vi "CRYPlot Octave Graph.vi"(6 "sOption":string, 7 "pGraph VI In":refnum<vi>, 9 "Flattened Property":string, 10 "Flattened Scale Property":string, 11 "Selected Rows In":i32[](array[numeric])) -> (0 "Color Info":u32[](array[numeric]), 1 "Curve Name":string[](array[string]), 2 "All Rows Out":i32[](array[numeric]), 3 "ItemSyms":i32[](array[numeric]))   [LabVIEW 2013]
uses:
  CRYWindow/DataView/Control/CRYGraph Scale.ctl
panel:
  in  "Graph Scale Property":T1={"X Scale.Maximum"=0.0, "X Scale.Minimum"=0.0, "Y0 Scale.Maximum"=0.0, "Y0 Scale.Minimum"=0.0, "Y1 Scale.Maximum"=0.0, "Y1 Scale.Minimum"=0.0, "X Scale.MapMode"=2, "Y1 Scale.MapMode"=2, "Y0 Scale.MapMode"=2, "ScaleFitX"=FALSE, "ScaleFitY"=FALSE, "ScaleFitY 2"=FALSE}
  in  "Plot Settings":T2(array[cluster])
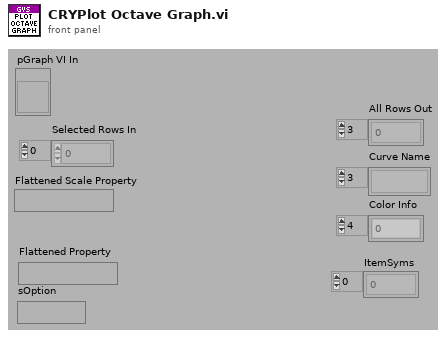
[diagram p1: front panel]
types:
  T1 = typedef "CRYGraph Scale.ctl" = cluster{"X Scale.Maximum":dbl, "X Scale.Minimum":dbl, "Y0 Scale.Maximum":dbl, "Y0 Scale.Minimum":dbl, "Y1 Scale.Maximum":dbl, "Y1 Scale.Minimum":dbl, "X Scale.MapMode":u8, "Y1 Scale.MapMode":u8, "Y0 Scale.MapMode":u8, "ScaleFitX":bool, "ScaleFitY":bool, "ScaleFitY 2":bool}
  T2 = cluster{"Color":u32, "Interpolation":u8, "Point Style":u8, "Line Style":u8, "Point Color":u32, "Line Width":u8, "Bar Plot Style":u8, "Fill To":i16}[]
  T3 = typedef "CRYData Cluster.ctl" = cluster{"Name":string, "Curve":cluster{"x":dbl, "y":dbl, "z":dbl}[], "X data":u16, "Y data":u16, "Z data":u16, "X axis":u16, "Y axis":u16, "Z axis":u16, "X unit":string, "Y unit":string, "Z unit":string, "X dB ref":dbl, "Y dB ref":dbl, "Z dB ref":dbl, "single val":bool, "protected":bool, "display X":bool, "display Y":bool, "display Z":bool, "Test Info":string, "Step No.":i32, "Plot Settings":cluster{"Color":u32, "Interpolation":u8, "Point Style":u8, "Line Style":u8, "Point Color":u32, "Line Width":u8, "Bar Plot Style":u8, "Fill To":i16}, "AutoProtect":bool}
  T4 = cluster{"Color":u32, "Interpolation":u8, "Point Style":u8, "Line Style":u8, "Point Color":u32, "Line Width":u8, "Bar Plot Style":u8, "Fill To":i16}
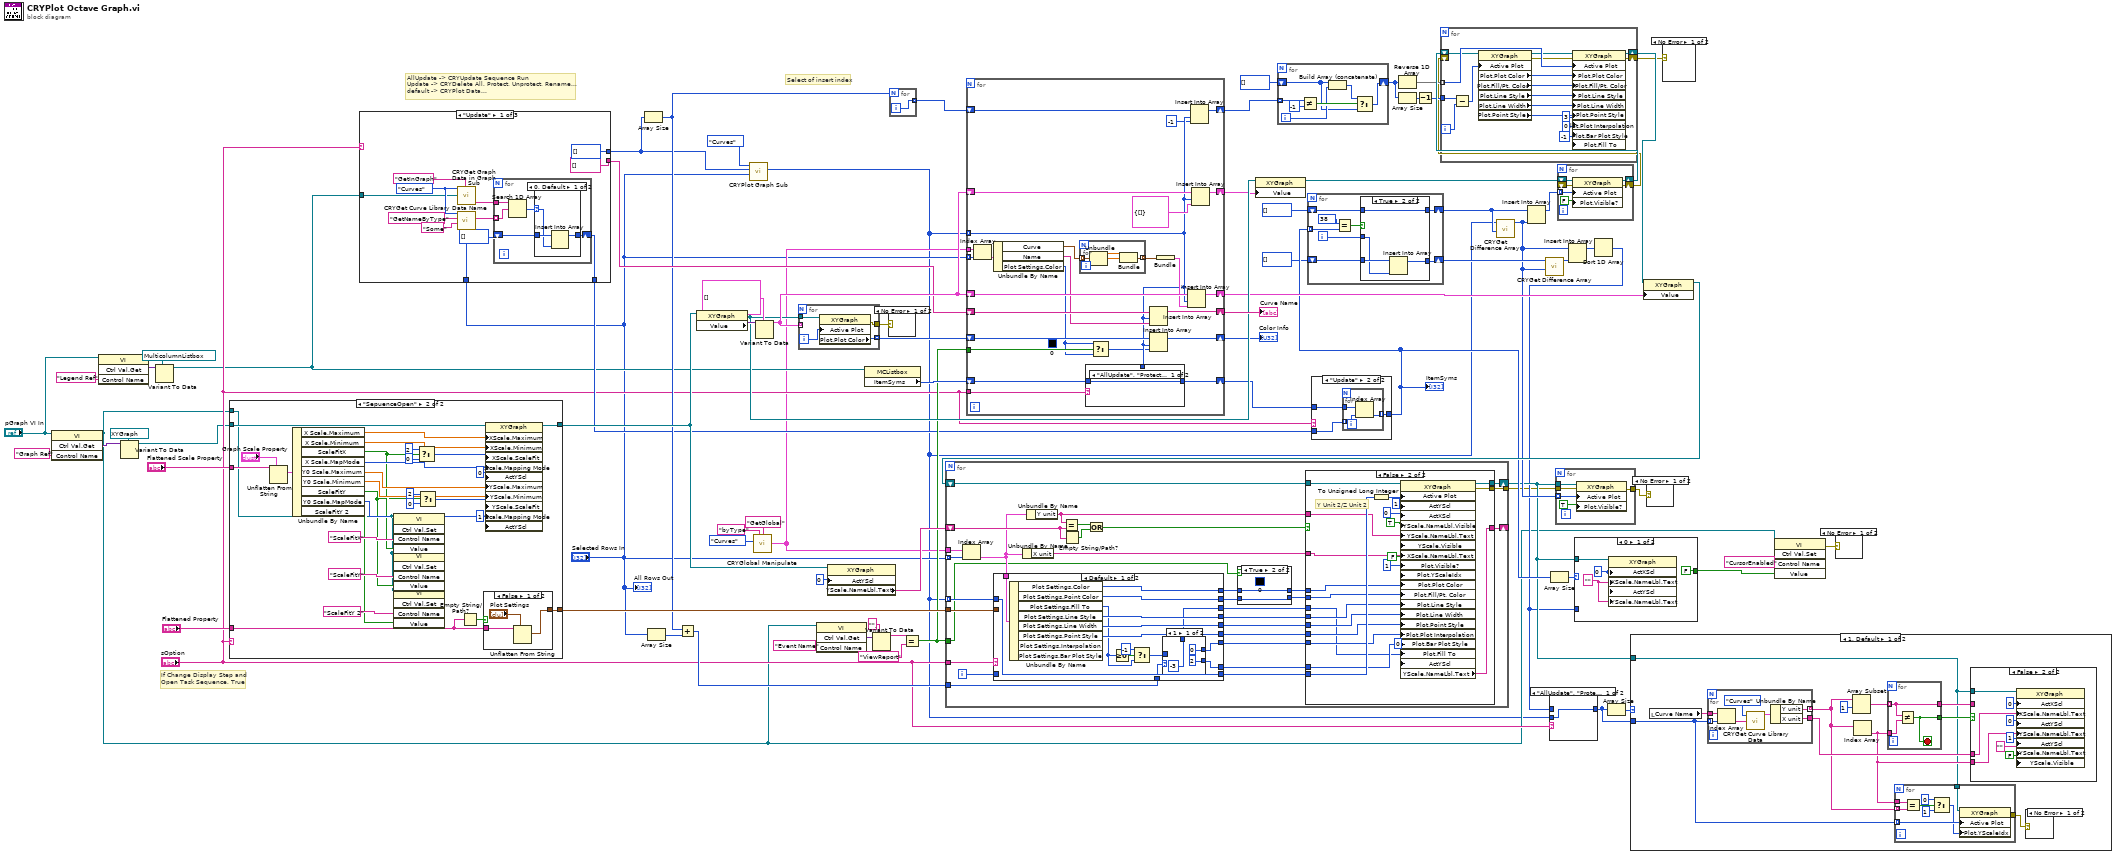
[diagram p0: block diagram]
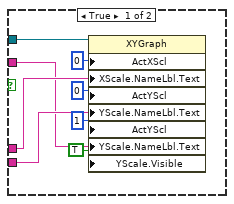
[diagram p7: hidden frame]
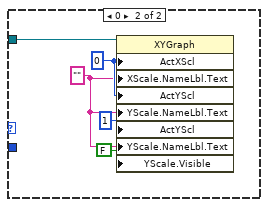
[diagram p8: hidden frame]
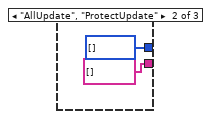
[diagram p11: hidden frame]
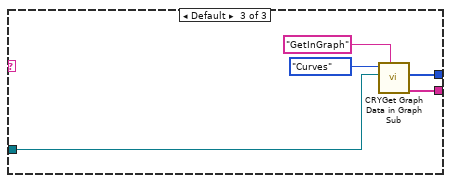
[diagram p12: hidden frame]
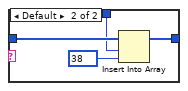
[diagram p13: hidden frame]
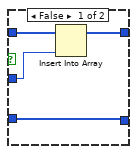
[diagram p15: hidden frame]
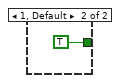
[diagram p16: hidden frame]
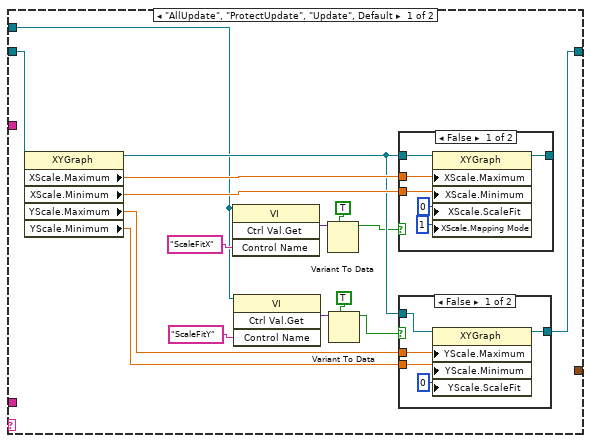
[diagram p17: hidden frame]
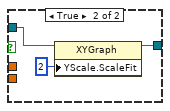
[diagram p18: hidden frame]
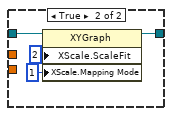
[diagram p19: hidden frame]
diagram:
  # "AllUpdate -> CRYUpdate Sequence Run\nUpdate -> CRYDelete All, Protect, Unprotect, Rename...\ndefault -> CRYPlot Data..."
  # "Select of insert index"
  # "If Change Display Step and \nOpen Task Sequence, True"
  n1 = invoke class="VI" method="Ctrl Val.Get"(reference="pGraph VI In", "Control Name"="Graph Ref") -> (reference out=w9:refnum<vi>, "Get Control Value Variant"=w13:variant)  [unwired: 2 in, 2 out]
  n2 = invoke class="VI" method="Ctrl Val.Get"(reference="pGraph VI In", "Control Name"="Legend Ref") -> ("Get Control Value Variant"=w17:variant)  [unwired: 2 in, 3 out]
  n3 = Variant To Data(type=refnum<vi> refnum ("XY Graph"), Variant=w13) -> (data=w12:refnum<vi>)  [unwired: 1 in, 1 out]
  n4 = Variant To Data(type=refnum<vi> refnum ("GMListbox"), Variant=w17) -> (data=w10:refnum<vi>)  [unwired: 1 in, 1 out]
  n5 = case shown="\"SepuenceOpen\"" "sOption" {
    tunnel: w12 -> [w96 w143]
    tunnel: [w91 w142] -> w59
    tunnel: "Flattened Scale Property" -> [_ w133]
    tunnel: [_ w129] -> w71
    tunnel: "Flattened Property" -> [_ w128]
    tunnel: w9 -> [w81 w115]
    frame "AllUpdate", "ProtectUpdate", "Update", Default {
      n6 = property class="XYGraph"(reference=w96) -> (reference out=w90:refnum<vi>, "XScale.Maximum"=w95:dbl, "XScale.Minimum"=w94:dbl, "YScale.Maximum"=w93:dbl, "YScale.Minimum"=w92:dbl)  [unwired: 1 in, 1 out]
      n7 = invoke class="VI" method="Ctrl Val.Get"(reference=w81, "Control Name"="ScaleFitX") -> ("Get Control Value Variant"=w85:variant)  [unwired: 2 in, 3 out]
      n8 = invoke class="VI" method="Ctrl Val.Get"(reference=w81, "Control Name"="ScaleFitY") -> ("Get Control Value Variant"=w88:variant)  [unwired: 2 in, 3 out]
      n9 = Variant To Data(type=TRUE, Variant=w85) -> (data=w83:bool)  [unwired: 1 in, 1 out]
      n10 = Variant To Data(type=TRUE, Variant=w88) -> (data=w82:bool)  [unwired: 1 in, 1 out]
      n11 = case shown="False" w83 {
        tunnel: w95 -> [w110 _]
        tunnel: w94 -> [w109 _]
        tunnel: w90 -> [w108 w114]
        tunnel: [w107 w113] -> _
        frame False {
          n12 = property class="XYGraph"(reference=w108, "XScale.Maximum"=w110, "XScale.Minimum"=w109, "XScale.ScaleFit"=u8 0 ("X Scale.Scale Fit"), "XScale.Mapping Mode"=u8 1 ("X Scale.Mapping Mode")) -> (reference out=w107:refnum<vi>)  [unwired: 1 in, 1 out]
        }
        frame True {
          n13 = property class="XYGraph"(reference=w114, "XScale.ScaleFit"=u8 2 ("X Scale.Scale Fit"), "XScale.Mapping Mode"=u8 1 ("X Scale.Mapping Mode")) -> (reference out=w113:refnum<vi>)  [unwired: 1 in, 1 out]
        }
      }
      n14 = case shown="False" w82 {
        tunnel: w90 -> [w101 w104]
        tunnel: [w100 w103] -> w91
        tunnel: w93 -> [w99 _]
        tunnel: w92 -> [w98 _]
        frame False {
          n15 = property class="XYGraph"(reference=w101, "YScale.Maximum"=w99, "YScale.Minimum"=w98, "YScale.ScaleFit"=u8 0 ("Y Scale.Scale Fit")) -> (reference out=w100:refnum<vi>)  [unwired: 1 in, 1 out]
        }
        frame True {
          n16 = property class="XYGraph"(reference=w104, "YScale.ScaleFit"=u8 2 ("Y Scale.Scale Fit")) -> (reference out=w103:refnum<vi>)  [unwired: 1 in, 1 out]
        }
      }
    }
    frame "SepuenceOpen" {
      n17 = Unflatten From String(type="Graph Scale Property", binary string=w133) -> (value=w132:T1)  [unwired: 3 in, 2 out]
      n18 = Unbundle By Name(w132) -> ("X Scale.Maximum"=w139:dbl, "X Scale.Minimum"=w138:dbl, "ScaleFitX"=w118:bool, "X Scale.MapMode"=w135:u8, "Y0 Scale.Maximum"=w137:dbl, "Y0 Scale.Minimum"=w136:dbl, "ScaleFitY"=w117:bool, "Y0 Scale.MapMode"=w134:u8, "ScaleFitY 2"=w116:bool)
      n19 = invoke class="VI" method="Ctrl Val.Set"(reference=w115, "Control Name"="ScaleFitX", "Value"=w118) -> ()  [unwired: 2 in, 5 out]
      n20 = invoke class="VI" method="Ctrl Val.Set"(reference=w115, "Control Name"="ScaleFitY", "Value"=w117) -> ()  [unwired: 2 in, 5 out]
      n21 = invoke class="VI" method="Ctrl Val.Set"(reference=w115, "Control Name"="ScaleFitY 2", "Value"=w116) -> ()  [unwired: 2 in, 5 out]
      n22 = Select(t=u8 2, s=w118, f=u8 0 ("X Scale.Scale Fit")) -> (s? t:f=w123:u8)
      n23 = Select(t=u8 2, s=w117, f=u8 0 ("X Scale.Scale Fit")) -> (s? t:f=w122:u8)
      n24 = Empty String/Path?(string/path=w128) -> (empty?=w130:bool)
      n25 = case shown="False" w130 {
        tunnel: w128 -> [w146 _]
        tunnel: [w144 _] -> w129
        frame False {
          n26 = Unflatten From String(type="Plot Settings", binary string=w146) -> (value=w144:T2)  [unwired: 3 in, 2 out]
        }
        frame True {
        }
      }
      n27 = property class="XYGraph"(reference=w143, "XScale.Maximum"=w139, "XScale.Minimum"=w138, "XScale.ScaleFit"=w123, "XScale.Mapping Mode"=w135, "ActYScl"=0 ("Active Y Scale"), "YScale.Maximum"=w137, "YScale.Minimum"=w136, "YScale.ScaleFit"=w122, "YScale.Mapping Mode"=w134, "ActYScl"=1 ("Active Y Scale")) -> (reference out=w142:refnum<vi>)  [unwired: 1 in, 1 out]
    }
  }
  n28 = case shown="\"Update\"" "sOption" {
    tunnel: [string[] [] ("Names Out") string[] [] ("Names Out") w174] -> w69
    tunnel: [i32[] [] ("Rows") i32[] [] ("Rows") w171] -> w3
    tunnel: "Selected Rows In" -> [w149 _ _]
    tunnel: [w148 _ _] -> w34
    tunnel: w10 -> [w147 _ w170]
    frame "Update" {
      w151 = enum16{"Curves", "Values", "Results", "WFM"}."Curves" ("Type")
      n29 = call "CRYGet Curve Library Data Name.vi"("nData"=w149, "sOption"="Some", "sAction"="GetNameByType", "Type"=w151) -> ("sNames"=w155:string[])  [unwired: 4 in, 3 out]
      n30 = call "CRYGet Graph Data in Graph Sub.vi"("sOption"="GetInGraph", "Legend Refnum"=w147, "Type In"=w151) -> ("Names Out"=w154:string[])  [unwired: 4 in, 4 out]
      n31 = for {
        tunnel: w154 -> [w160]
        tunnel: w155 -> [w159] mode=indexing
        shift-right: [w161] -> w148
        shift-left: i32[] [] -> [w162]
        n32 = Search 1D Array(1D array=w160, element=w159) -> (index of element=w163:i32)  [unwired: 1 in]
        n33 = case shown="0, Default" w163 {
          selector: w163 -> [w164 _]
          tunnel: w162 -> [w166 w167]
          tunnel: [w165 w167] -> w161
          frame 0, Default {
            n34 = Insert Into Array(array=w166, new element=w164) -> (w165:i32[])  [unwired: 1 in]
          }
          frame -1 {
          }
        }
      }
    }
    frame "AllUpdate", "ProtectUpdate" {
    }
    frame Default {
      n35 = call "CRYGet Graph Data in Graph Sub.vi"("sOption"="GetInGraph", "Legend Refnum"=w170, "Type In"=enum16{"Curves", "Values", "Results", "WFM"}."Curves" ("Type")) -> ("Names Out"=w174:string[], "Rows"=w171:i32[])  [unwired: 4 in, 3 out]
    }
  }
  n36 = Array Size(array=w3) -> (size(s)=w39:i32)
  n37 = Array Size(array="Selected Rows In") -> (size(s)=w40:i32)
  n38 = Add(x=w39, y=w40) -> (x+y=w38:i32)
  n39 = property class="XYGraph"(reference=w59) -> (reference out=w67:refnum<vi>, "Value"=w77:variant)  [unwired: 1 in, 1 out]
  n40 = call "CRYPlot Graph Sub.vi"("nData2 In"="Selected Rows In", "nData1 In"=w3, "Type"=enum16{"Curves", "Values", "Results", "WFM"}."Curves") -> ("nData Out"=w1:i32[])  [unwired: 8 in]
  n41 = call "CRYGlobal Manipulate.vi"("Type"=enum16{"Curves", "Values", "Results", "WFM"}."Curves", "sOption"="byType", "sAction"="GetGlobal") -> ("Curves Out"=w5:T3[])  [unwired: 6 in, 6 out]
  n42 = Variant To Data(type=cluster{cluster{"x":dbl, "z":dbl}[]}[] [], Variant=w77) -> (data=w76:cluster{cluster{"x":dbl, "z":dbl}[]}[])  [unwired: 1 in, 1 out]
  n43 = for {
    tunnel: w76 -> [_] mode=indexing
    tunnel: w67 -> [w178]
    tunnel: [w177] -> w75 mode=indexing
    tunnel: [w175] -> w20
    i -> [w176]
    n44 = property class="XYGraph"(reference=w178, "Active Plot"=w176) -> (error out=w175:errorcluster, "Plot.Plot Color"=w177:u32)  [unwired: 1 in, 1 out]
  }
  n45 = invoke class="VI" method="Ctrl Val.Get"(reference=w9, "Control Name"="Event Name") -> ("Get Control Value Variant"=w46:variant)  [unwired: 2 in, 3 out]
  n46 = property class="XYGraph"(reference=w59, "ActYScl"=0 ("Active Y Scale")) -> ("YScale.NameLbl.Text"=w60:string)  [unwired: 1 in, 2 out]
  n47 = property class="MCListbox"(reference=w10) -> ("ItemSyms"=w63:i32[])  [unwired: 1 in, 2 out]
  n48 = Variant To Data(type="" ("Control Name"), Variant=w46) -> (data=w44:string)  [unwired: 1 in, 1 out]
  n49 = case shown="No Error" w20 {
    frame No Error {
    }
    frame Error {
    }
  }
  n50 = for {
    N: w39 -> [_]
    tunnel: [w179] -> w57 mode=indexing
    i -> [w179]
  }
  n51 = Equal?(x=w44, y="ViewReport" ("regular expression")) -> (x = y?=w42:bool)
  n52 = for {
    tunnel: w5 -> [w205]
    tunnel: "Selected Rows In" -> [w202] mode=indexing
    shift-right: [w203] -> w65
    shift-left: w76 -> [w204]
    tunnel: w1 -> [w185] mode=indexing
    shift-right: [w193] -> w74
    shift-left: w69 -> [w197]
    shift-right: [w194] -> w41
    shift-left: w75 -> [w195]
    shift-right: [w191] -> w64
    shift-left: w76 -> [w190]
    shift-right: [w188] -> w35
    shift-left: w63 -> [w189]
    shift-right: [w186] -> w56
    shift-left: w57 -> [w187]
    tunnel: w42 -> [w183]
    tunnel: "sOption" -> [w181]
    (unwired) u32 0
    n53 = Index Array(array=w205, index=w202) -> (element=w199:T3)
    n54 = Unbundle By Name(w199) -> ("Curve"=w200:cluster{"x":dbl, "y":dbl, "z":dbl}[], "Name"=w196:string, "Plot Settings.Color"=w180:u32)
    n55 = for {
      tunnel: w200 -> [w213] mode=indexing
      tunnel: [w212] -> w201 mode=indexing
      n56 = Unbundle(w213) -> ("x"=w211:dbl, "y"=w214:dbl)  [unwired: 1 out]
      n57 = Bundle("x"=w211, "y"=w214) -> (w212:cluster{"x":dbl, "y":dbl})  [unwired: 1 out]
    }
    n58 = case shown="\"AllUpdate\", \"ProtectUpdate\", \"Update\"" w181 {
      tunnel: w189 -> [w206 w210]
      tunnel: [w206 w209] -> w188
      tunnel: w185 -> [_ w207]
      frame "AllUpdate", "ProtectUpdate", "Update" {
      }
      frame Default {
        n59 = Insert Into Array(array=w210, index=w207, new element=38) -> (w209:i32[])
      }
    }
    n60 = Select(t=w180, s=w183, f=w180) -> (s? t:f=w182:u32)
    n61 = Insert Into Array(array=w197, index=w185, new element=w196) -> (w193:string[])
    n62 = Insert Into Array(array=w195, index=w185, new element=w182) -> (w194:u32[])
    n63 = Bundle(w201) -> (w198:cluster{cluster{"x":dbl, "y":dbl}[]})  [unwired: 1 in]
    n64 = Insert Into Array(array=w204, index=w185, new element=w198) -> (w203:cluster{cluster{"x":dbl, "z":dbl}[]}[])
    n65 = Insert Into Array(array=w187, index=w185, new element=-1 ("new element/subarray")) -> (w186:i32[])
    n66 = Insert Into Array(array=w190, index=w185, new element=cluster{cluster{"x":dbl, "y":dbl}[]} {[]} ("output cluster")) -> (w191:cluster{cluster{"x":dbl, "z":dbl}[]}[])
  }
  "Curve Name" <- w74
  "Color Info" <- w41
  n67 = property class="XYGraph"(reference=w67, "Value"=w64) -> (reference out=w66:refnum<vi>)  [unwired: 1 in, 1 out]
  n68 = for {
    tunnel: w56 -> [w221] mode=indexing
    shift-right: [w217] -> w51
    shift-left: i32[] [] ("Selected Rows In") -> [w215]
    i -> [w216]
    n69 = Not Equal?(x=w221, y=-1) -> (x != y?=w219:bool)
    n70 = Build Array (concatenate)(w215, w216) -> (w218:i32[])
    n71 = Select(t=w218, s=w219, f=w215) -> (s? t:f=w217:i32[])
  }
  n72 = case shown="\"Update\"" "sOption" {
    tunnel: w34 -> [_ w224]
    tunnel: w35 -> [w222 w225]
    tunnel: [w222 w223] -> w33
    frame Default {
    }
    frame "Update" {
      n73 = for {
        tunnel: w225 -> [w228]
        tunnel: w224 -> [w227] mode=indexing
        tunnel: [w226] -> w223 mode=indexing
        n74 = Index Array(array=w228, index=w227) -> (element=w226:i32)
      }
    }
  }
  "ItemSyms" <- w33
  n75 = for {
    tunnel: w33 -> [w235] mode=indexing
    shift-right: [w234] -> w37
    shift-left: i32[] [] ("Selected Rows In") -> [w233]
    shift-right: [w229] -> w29
    shift-left: i32[] [] ("Selected Rows In") -> [w230]
    i -> [w232]
    n76 = Equal?(x=38, y=w235) -> (x = y?=w231:bool)
    n77 = case shown="True" w231 {
      tunnel: [w239 w241] -> w234
      tunnel: w233 -> [w240 w241]
      tunnel: w232 -> [w238 w242]
      tunnel: w230 -> [w237 w244]
      tunnel: [w237 w243] -> w229
      frame False {
        n78 = Insert Into Array(array=w240, new element=w238) -> (w239:i32[])  [unwired: 1 in]
      }
      frame True {
        n79 = Insert Into Array(array=w244, new element=w242) -> (w243:i32[])  [unwired: 1 in]
      }
    }
  }
  n80 = Reverse 1D Array(array=w51) -> (reversed array=w52:i32[])
  n81 = Array Size(array=w51) -> (size(s)=w50:i32)
  n82 = Decrement(x=w50) -> (x-1=w49:i32)
  n83 = call "CRYGet Difference Array.vi"("Array 2"=w37, "Array 1"=w1) -> ("Diff Out"=w28:i32[])  [unwired: 8 in, 1 out]
  n84 = Insert Into Array(array=w37, new element=w28) -> (w58:i32[])  [unwired: 1 in]
  n85 = call "CRYGet Difference Array.vi"("Array 2"=w28, "Array 1"=w29) -> ("Diff Out"=w31:i32[])  [unwired: 8 in, 1 out]
  n86 = Array Size(array=w33) -> (size(s)=w80:i32)
  n87 = for {
    shift-right: [w248] -> w54
    shift-left: w66 -> [w250]
    tunnel: w58 -> [w247] mode=indexing
    shift-right: [w246] -> w36
    shift-left: _ -> [w245]
    n88 = property class="XYGraph"(reference=w250, error in=w245, "Active Plot"=w247, "Plot.Visible?"=FALSE ("Plot.Visible")) -> (reference out=w248:refnum<vi>, error out=w246:errorcluster)
  }
  n89 = for {
    tunnel: w52 -> [w262] mode=indexing
    shift-right: [w260] -> w53
    shift-left: w54 -> [w261]
    tunnel: w49 -> [w258]
    shift-right: [w254] -> w48
    shift-left: w36 -> [_]
    i -> [w257]
    n90 = Subtract(x=w258, y=w257) -> (x-y=w256:i32)
    n91 = property class="XYGraph"(reference=w261, "Active Plot"=w256) -> (reference out=w259:refnum<vi>, error out=w255:errorcluster, "Plot.Plot Color"=w267:u32, "Plot.Fill/Pt. Color"=w266:u32, "Plot.Line Style"=w265:u8, "Plot.Line Width"=w264:u8, "Plot.Point Style"=w263:u8)  [unwired: 1 in]
    n92 = property class="XYGraph"(reference=w259, error in=w255, "Active Plot"=w262, "Plot.Plot Color"=w267, "Plot.Fill/Pt. Color"=w266, "Plot.Line Style"=w265, "Plot.Line Width"=w264, "Plot.Point Style"=w263, "Plot.Plot Interpolation"=u8 3, "Plot.Bar Plot Style"=u8 0, "Plot.Fill To"=i16 -1) -> (reference out=w260:refnum<vi>, error out=w254:errorcluster)
  }
  n93 = Insert Into Array(array=w28, new element=w31) -> (w30:i32[])  [unwired: 1 in]
  n94 = Sort 1D Array(array=w30) -> (sorted array=w24:i32[])
  n95 = case shown="\"AllUpdate\", \"ProtectUpdate\", \"SepuenceOpen\"" "sOption" {
    tunnel: [w268 w269] -> w23
    tunnel: w1 -> [w268 _]
    tunnel: w24 -> [_ w269]
    frame "AllUpdate", "ProtectUpdate", "SepuenceOpen" {
    }
    frame Default {
    }
  }
  n96 = Array Size(array=w23) -> (size(s)=w27:i32)
  n97 = property class="XYGraph"(reference=w53, "Value"=w65) -> (reference out=w73:refnum<vi>)  [unwired: 1 in, 1 out]
  n98 = for {
    tunnel: "Selected Rows In" -> [w299] mode=indexing
    tunnel: w5 -> [w298]
    tunnel: w71 -> [w293]
    tunnel: "sOption" -> [w294]
    shift-right: [w295] -> w26
    shift-left: w73 -> [w283]
    tunnel: w1 -> [w282] mode=indexing
    shift-right: [w280] -> _
    shift-left: w60 -> [w286]
    tunnel: w42 -> [w278]
    tunnel: w38 -> [w271]
    tunnel: [w270] -> w19
    i -> [w287]
    n99 = Index Array(array=w298, index=w299) -> (element=w285:T3)
    n100 = case shown="Default" w294 {
      tunnel: w293 -> [_ w330]
      tunnel: [w318 w339] -> w277
      tunnel: [w317 w338] -> w275
      tunnel: [w305 w327] -> w292
      tunnel: [w316 w337] -> w291
      tunnel: [w315 w336] -> w290
      tunnel: [w314 w335] -> w289
      tunnel: [w307 w326] -> w288
      tunnel: w285 -> [w313 _]
      tunnel: w287 -> [_ w329]
      tunnel: [w309 w331] -> w281
      tunnel: w282 -> [w309 w331]
      tunnel: [w306 w325] -> w279
      tunnel: w271 -> [w308 _]
      frame Default {
        n101 = Unbundle By Name(w313) -> ("Plot Settings.Color"=w318:u32, "Plot Settings.Point Color"=w317:u32, "Plot Settings.Fill To"=w310:i16, "Plot Settings.Line Style"=w316:u8, "Plot Settings.Line Width"=w315:u8, "Plot Settings.Point Style"=w314:u8)  [unwired: 2 out]
        n102 = Greater Or Equal To 0?(x=w310) -> (x >= 0?=w312:bool)
        n103 = Select(t=i16 -1 ("Fill To"), s=w312, f=w310) -> (s? t:f=w304:i16)
        n104 = case shown="1" w308 {
          tunnel: [u8 2 u8 0] -> w306
          tunnel: [u8 0 u8 3] -> w307
          tunnel: [i16 -3 ("Fill To") i16 -1 ("Fill To")] -> w305
          tunnel: w304 -> [_ _]
          frame 1 {
          }
          frame 2, Default {
          }
        }
      }
      frame "SepuenceOpen" {
        n105 = Index Array(array=w330, index=w329) -> (element=w328:T4)
        n106 = Unbundle By Name(w328) -> ("Color"=w339:u32, "Point Color"=w338:u32, "Fill To"=w332:i16, "Line Style"=w337:u8, "Line Width"=w336:u8, "Point Style"=w335:u8, "Interpolation"=w326:u8, "Bar Plot Style"=w325:u8)
        n107 = Greater Or Equal To 0?(x=w332) -> (x >= 0?=w334:bool)
        n108 = Select(t=i16 -1 ("Fill To"), s=w334, f=w332) -> (s? t:f=w327:i16)
      }
    }
    n109 = Unbundle By Name(w285) -> ("X unit"=w284:string)
    n110 = Unbundle By Name(w285) -> ("Y unit"=w296:string)
    n111 = Equal?(x=w296, y=w286) -> (x = y?=w272:bool)
    n112 = Empty String/Path?(string/path=w286) -> (empty?=w273:bool)
    n113 = Or(x=w272, y=w273) -> (x .or. y?=w297:bool)
    n114 = case shown="True" w278 {
      tunnel: [w301 w303] -> w276
      tunnel: w277 -> [w301 w303]
      tunnel: w275 -> [w300 w302]
      tunnel: [w300 w302] -> w274
      frame False {
      }
      frame True {
        (unwired) u32 0
      }
    }
    n115 = case shown="False" w297 {
      tunnel: w284 -> [w349 w359]
      tunnel: w283 -> [w357 w378]
      tunnel: w281 -> [w356 w379]
      tunnel: w296 -> [w344 w364]
      tunnel: [w355 w377] -> w295
      tunnel: w276 -> [w354 w376]
      tunnel: w274 -> [w342 w375]
      tunnel: w292 -> [w341 w360]
      tunnel: w291 -> [w353 w374]
      tunnel: w290 -> [w352 w373]
      tunnel: w289 -> [w351 w372]
      tunnel: w288 -> [w350 w371]
      tunnel: [w344 w362] -> w280
      tunnel: w279 -> [w343 w361]
      tunnel: [w340 w358] -> w270
      frame True {
        w346 = 0 ("Active X Scale")
        # "Y Unit 1/Z Unit 1"
        n116 = To Unsigned Long Integer(number=w356) -> (unsigned 32bit integer=w345:u32)
        n117 = property class="XYGraph"(reference=w357, "Active Plot"=w345, "ActXScl"=w346, "XScale.NameLbl.Text"=w349, "ActYScl"=w346, "YScale.NameLbl.Text"=w344, "Plot.Visible?"=FALSE ("Plot.Visible"), "Plot.YScaleIdx"=u32 0 ("Plot.Y Scale Index"), "Plot.Plot Color"=w354, "Plot.Fill/Pt. Color"=w342, "Plot.Line Style"=w353, "Plot.Line Width"=w352, "Plot.Point Style"=w351, "Plot.Plot Interpolation"=w350, "Plot.Bar Plot Style"=w343, "Plot.Fill To"=w341) -> (reference out=w355:refnum<vi>, error out=w340:errorcluster)  [unwired: 1 in]
      }
      frame False {
        w367 = TRUE ("Y Scale.Name Label.Visible")
        # "Y Unit 2/Z Unit 2"
        n118 = To Unsigned Long Integer(number=w379) -> (unsigned 32bit integer=w366:u32)
        n119 = property class="XYGraph"(reference=w378, "Active Plot"=w366, "ActYScl"=1 ("Active Y Scale"), "ActXScl"=0 ("Active X Scale"), "YScale.NameLbl.Visible"=w367, "YScale.NameLbl.Text"=w364, "YScale.Visible"=w367, "XScale.NameLbl.Text"=w359, "Plot.Visible?"=FALSE ("Plot.Visible"), "Plot.YScaleIdx"=u32 1 ("Plot.Y Scale Index"), "Plot.Plot Color"=w376, "Plot.Fill/Pt. Color"=w375, "Plot.Line Style"=w374, "Plot.Line Width"=w373, "Plot.Point Style"=w372, "Plot.Plot Interpolation"=w371, "Plot.Bar Plot Style"=w361, "Plot.Fill To"=w360, "ActYScl"=0 ("Active Y Scale")) -> (reference out=w377:refnum<vi>, error out=w358:errorcluster, "YScale.NameLbl.Text"=w362:string)  [unwired: 1 in]
      }
    }
  }
  n120 = for {
    tunnel: w26 -> [w384]
    tunnel: w28 -> [w382] mode=indexing
    tunnel: [w381] -> w21
    tunnel: w19 -> [w380]
    n121 = property class="XYGraph"(reference=w384, error in=w380, "Active Plot"=w382, "Plot.Visible?"=TRUE ("Plot.Visible")) -> (error out=w381:errorcluster)  [unwired: 1 out]
  }
  n122 = case shown="0" w80 {
    tunnel: w26 -> [w386 _]
    tunnel: [FALSE TRUE] -> w79
    tunnel: w24 -> [_ _]
    frame 0 {
      w388 = 0 ("Active X Scale")
      w387 = "" ("X Scale.Name Label.Text")
      n123 = property class="XYGraph"(reference=w386, "ActXScl"=w388, "XScale.NameLbl.Text"=w387, "ActYScl"=w388, "YScale.NameLbl.Text"=w387) -> ()  [unwired: 1 in, 2 out]
    }
    frame 1, Default {
    }
  }
  n124 = case shown="1, Default" w27 {
    tunnel: w23 -> [w392 _]
    tunnel: w26 -> [w391 w439]
    frame 1, Default {
      n125 = local read "Curve Name"() -> (w400:string[])
      n126 = for {
        tunnel: w400 -> [w434]
        tunnel: w392 -> [w435] mode=indexing
        tunnel: [w430] -> w394 mode=indexing
        tunnel: [w429] -> w396
        n127 = Index Array(array=w434, index=w435) -> (element=w433:string)
        n128 = call "CRYGet Curve Library Data.vi"("Type"=enum16{"Curves", "Values", "Results", "WFM"}."Curves", "Data Name"=w433) -> ("Curve"=w431:T3)  [unwired: 4 out]
        n129 = Unbundle By Name(w431) -> ("Y unit"=w430:string, "X unit"=w429:string)
      }
      n130 = Array Subset(array=w394, index=1) -> (w398:string[])  [unwired: 1 in]
      n131 = Index Array(array=w394) -> (element=w393:string)  [unwired: 1 in]
      n132 = for {
        tunnel: w398 -> [w426] mode=indexing
        tunnel: w393 -> [w428]
        tunnel: [w427] -> w397
        tunnel: [w426] -> w395
        stop <- w427 stop-if-true
        n133 = Not Equal?(x=w426, y=w428) -> (x != y?=w427:bool)
      }
      n134 = for {
        tunnel: w392 -> [w409] mode=indexing
        tunnel: w394 -> [w407] mode=indexing
        tunnel: w393 -> [w408]
        tunnel: w391 -> [w402]
        tunnel: [w401] -> w390
        n135 = Equal?(x=w408, y=w407) -> (x = y?=w406:bool)
        n136 = Select(t=u32 0 ("Plot.Y Scale Index"), s=w406, f=u32 1 ("Plot.Y Scale Index")) -> (s? t:f=w403:u32)
        n137 = property class="XYGraph"(reference=w402, "Active Plot"=w409, "Plot.YScaleIdx"=w403) -> (error out=w401:errorcluster)  [unwired: 1 in, 1 out]
      }
      n138 = case shown="False" w397 {
        tunnel: w393 -> [w414 w422]
        tunnel: w396 -> [w413 w420]
        tunnel: w395 -> [w411 _]
        tunnel: w391 -> [w410 w418]
        frame True {
          n139 = property class="XYGraph"(reference=w410, "ActXScl"=0 ("Active X Scale"), "XScale.NameLbl.Text"=w413, "ActYScl"=0 ("Active X Scale"), "YScale.NameLbl.Text"=w414, "ActYScl"=1 ("Active Y Scale"), "YScale.NameLbl.Text"=w411, "YScale.Visible"=TRUE ("Y Scale.Visible")) -> ()  [unwired: 1 in, 2 out]
        }
        frame False {
          n140 = property class="XYGraph"(reference=w418, "ActXScl"=0 ("Active X Scale"), "XScale.NameLbl.Text"=w420, "ActYScl"=0 ("Active X Scale"), "YScale.NameLbl.Text"=w422, "ActYScl"=1 ("Active Y Scale"), "YScale.NameLbl.Text"="" ("Y Scale.Name Label.Text"), "YScale.Visible"=FALSE ("Y Scale.Visible")) -> ()  [unwired: 1 in, 2 out]
        }
      }
      n141 = case shown="No Error" w390 {
        frame No Error {
        }
        frame Error {
        }
      }
    }
    frame 0 {
      w440 = 0 ("Active X Scale")
      w437 = "" ("X Scale.Name Label.Text")
      n142 = property class="XYGraph"(reference=w439, "ActXScl"=w440, "XScale.NameLbl.Text"=w437, "ActYScl"=w440, "YScale.NameLbl.Text"=w437, "ActYScl"=1 ("Active Y Scale"), "YScale.NameLbl.Text"=w437, "YScale.Visible"=FALSE ("Y Scale.Visible")) -> ()  [unwired: 1 in, 2 out]
    }
  }
  n143 = case shown="No Error" w21 {
    frame No Error {
    }
    frame Error {
    }
  }
  n144 = case shown="No Error" w48 {
    frame No Error {
    }
    frame Error {
    }
  }
  n145 = invoke class="VI" method="Ctrl Val.Set"(reference=w9, "Control Name"="CursorEnabled", "Value"=w79) -> (error out=w22:errorcluster)  [unwired: 2 in, 4 out]
  n146 = case shown="No Error" w22 {
    frame No Error {
    }
    frame Error {
    }
  }
  "All Rows Out" <- "Selected Rows In"
